vi "Write.vi"(8 "error in (no error)":errorcluster caption="entrée d'erreur (pas d'erreur)", 11 "Class CSV_File (Default) en entrée":refnum<class "Class CSV_File.lvclass">) -> (0 "error out":errorcluster caption="sortie d'erreur", 3 "Class CSV_File (Default) en sortie":refnum<class "Class CSV_File.lvclass">)   [LabVIEW 2020, in "Library Instrument & Equipement.lvlib" / "Library File.lvlib" / "Class CSV_File.lvclass"]
uses:
  Class CSV_File.lvclass
  C:/Users/ngarcin/OneDrive - Altyor/Standard TB/Class/Read CSV File/Class File (Default)/Class File (Default).lvclass
  Class File (Default)/Class File (Default).lvclass
  Class CSV_File.lvclass/Class CSV_File.ctl
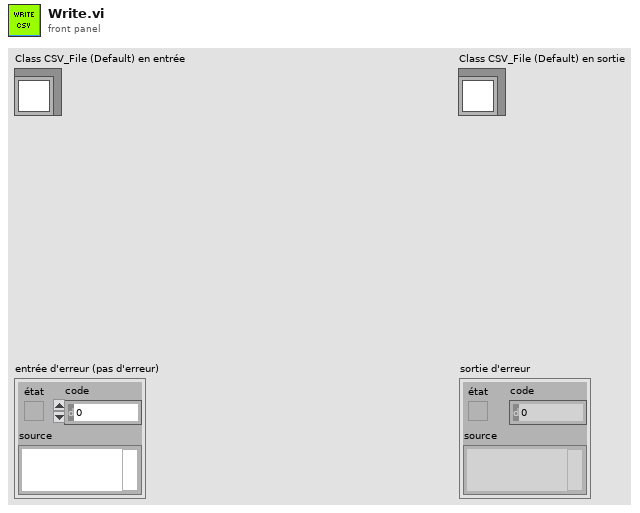
[diagram p1: front panel]
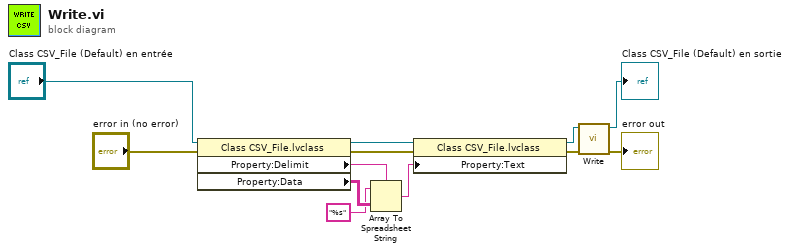
[diagram p0: block diagram]
diagram:
  n1 = property class="Class CSV_File.lvclass"(reference="Class CSV_File (Default) en entrée", error in="error in (no error)") -> (reference out=w6:refnum<class "Class CSV_File.lvclass">, error out=w2:errorcluster, "Property:Delimit"=w3:string, "Property:Data"=w5:string[][])
  n2 = Array To Spreadsheet String(delimiter (Tab)=w3, array=w5, 3:"%s" ("chaîne de format")) -> (spreadsheet string=w1:string)
  n3 = property class="Class CSV_File.lvclass"(reference=w6, error in=w2, "Property:Text"=w1) -> (reference out=w9:refnum<class "Class CSV_File.lvclass">, error out=w10:errorcluster)
  n4 = call-parent "Write.vi"("error in (no error)"=w10, "Class CSV_File (Default) en entrée"=w9) -> ("error out"=→"error out":errorcluster, "Class CSV_File (Default) en sortie"=→"Class CSV_File (Default) en sortie":refnum<class "Class CSV_File.lvclass">)  [unwired: 8 in]
